vi "FTW-Package-Compose.vi"(2 "Message Body":string, 3 "Message Header":string, 4 "Sender Identity":string) -> (0 "Multipart Message":string[](array[string]))   [LabVIEW 2013, in "FTW-Package.lvclass"]
uses:
  FTW-Package.lvclass
panel:
  # "Inputs"
  # "Outputs"
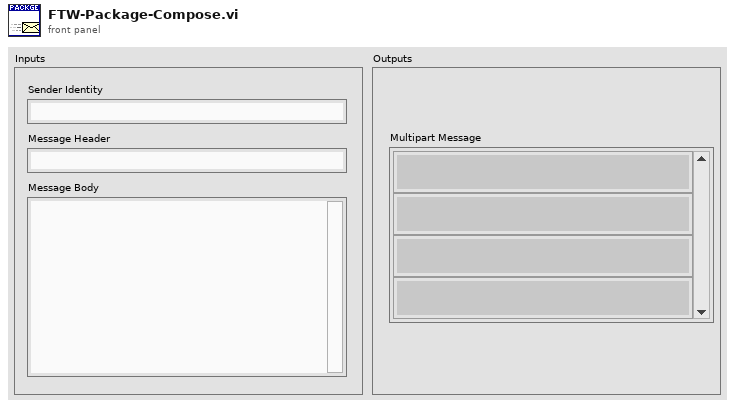
[diagram p1: front panel]
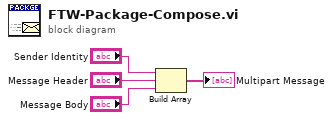
[diagram p0: block diagram]
diagram:
  n1 = Build Array("Sender Identity", "Message Header", "Message Body") -> (→"Multipart Message":string[])
